vi "UpDownNone.vi"(1 "Down":bool, 2 "Up":bool, 3 "x":dbl) -> (0 "Result":dbl)   [LabVIEW 2012]
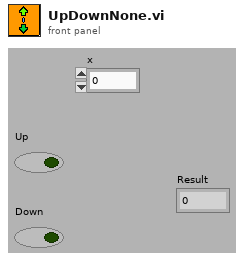
[diagram p1: front panel]
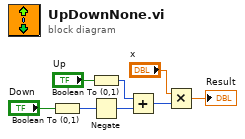
[diagram p0: block diagram]
diagram:
  n1 = Boolean To (0,1)(Boolean="Down") -> (0, 1=w5:i16)
  n2 = Boolean To (0,1)(Boolean="Up") -> (0, 1=w6:i16)
  n3 = Negate(x=w5) -> (-x=w1:i16)
  n4 = Add(x=w6, y=w1) -> (x+y=w4:i16)
  n5 = Multiply(x="x", y=w4) -> (x*y=→"Result":dbl)
